vi "Write To DBL File.vi"(4 "append to file? (new file:F)":bool, 5 "1D array":dbl[](array[numeric]) format="%0.2f", 7 "file path (dialog if empty)":path) -> (1 "new file path (Not A Path if cancelled)":path)   [LabVIEW 2010]
doc: "Writes a 2D or 1D array of single-precision numbers (SGL) to a new byte stream file or appends the data to an existing file."
panel:
  in  "prompt":string="Choose file to write."
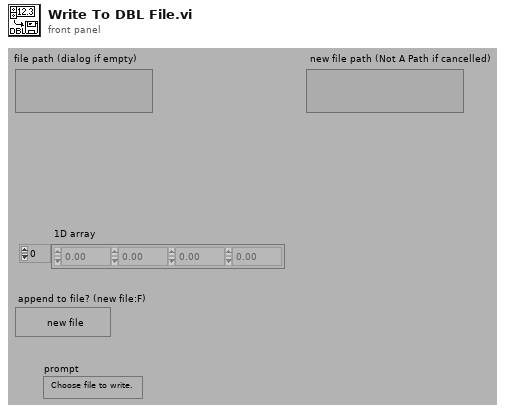
[diagram p1: front panel]
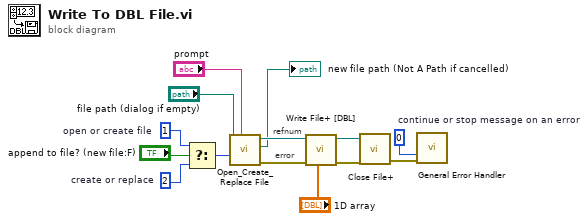
[diagram p0: block diagram]
diagram:
  w4 = i16 2  # create or replace
  w12 = 0  # continue or stop message on an error
  w7 = i16 1  # open or create file
  # "error"
  # "refnum"
  n1 = Select(t=w7, s="append to file? (new file:F)", f=w4) -> (s? t:f=w9:i16)
  n2 = call <vilib>:"Open_Create_Replace File.vi"("prompt"="prompt", "function (open:0)"=w9, "file path"="file path (dialog if empty)") -> ("error out"=w13:errorcluster, "new file path"=→"new file path (Not A Path if cancelled)":path, "refnum"=w3:refnum<file>)  [unwired: 5 in, 1 out]
  n3 = call "Write File+ [DBL].vi"("1D array"="1D array", "error in (no error)"=w13, "refnum"=w3) -> ("error out"=w11:errorcluster, "dup refnum"=w10:refnum<file>)  [unwired: 6 in, 1 out]
  n4 = call <vilib>:"Close File+.vi"("error in (no error)"=w11, "refnum"=w10) -> ("error out"=w8:errorcluster)  [unwired: 3 in, 2 out]
  n5 = call <vilib>:"General Error Handler.vi"("type of dialog (OK msg:1)"=w12, "error in (no error)"=w8) -> ()  [unwired: 9 in, 5 out]
